vi "Calculate Current Limit.vi"(9 "Voltage value":dbl, 10 "Maximum power":dbl, 11 "Current limit in":dbl) -> (3 "Current limit out":dbl)   [LabVIEW 2021, in "PMIC Common.lvlib"]
uses:
  PMIC Common.lvlib
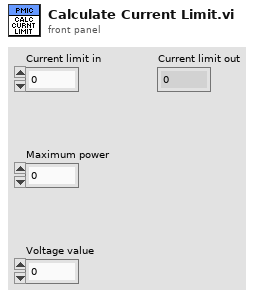
[diagram p1: front panel]
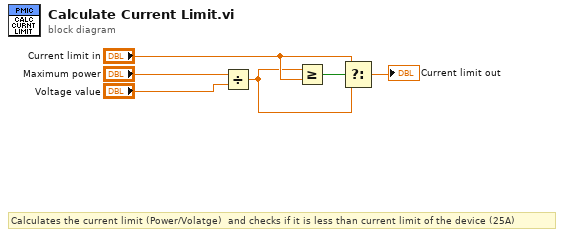
[diagram p0: block diagram]
diagram:
  # "Calculates the current limit (Power/Volatge)  and checks if it is less than current limit of the device (25A)"
  n1 = Divide(x="Maximum power", y="Voltage value") -> (x/y=w5:dbl)
  n2 = Greater Or Equal?(x=w5, y="Current limit in") -> (x >= y?=w4:bool)
  n3 = Select(t="Current limit in", s=w4, f=w5) -> (s? t:f=→"Current limit out":dbl)
